vi "generate_virtual_folder.vi"   [LabVIEW 2010]
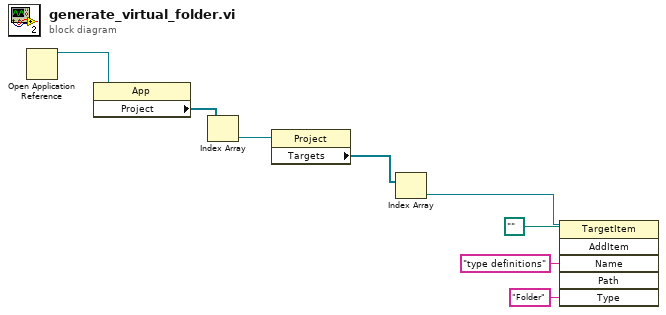
[diagram p0: block diagram]
diagram:
  n1 = Open Application Reference() -> (3:w8:refnum<vi>)  [unwired: 4 in, 1 out]
  n2 = property class="App"(reference=w8) -> ("Project"=w7:refnum<vi>[])  [unwired: 1 in, 2 out]
  n3 = Index Array(array=w7) -> (element=w6:refnum<vi>)  [unwired: 1 in]
  n4 = property class="Project"(reference=w6) -> ("Targets"=w5:refnum<vi>[])  [unwired: 1 in, 2 out]
  n5 = Index Array(array=w5) -> (element=w1:refnum<vi>)  [unwired: 1 in]
  n6 = invoke class="TargetItem" method="AddItem"(reference=w1, "Name"="type definitions", "Path"=path "", "Type"="Folder") -> ()  [unwired: 2 in, 6 out]
